vi "写入消息.vi"(8 "error in (no error)":errorcluster caption="错误输入（无错误）", 10 "操作者框架:消息待入队列":refnum<class "Message Enqueuer.lvclass">, 11 "用户操作输入":refnum<class "用户操作.lvclass">) -> (0 "error out":errorcluster caption="错误输出", 3 "用户操作输出":refnum<class "用户操作.lvclass">)   [LabVIEW 2020, in "用户操作.lvlib" / "用户操作.lvclass"]
uses:
  <vilib>/ActorFramework/Message Enqueuer/Message Enqueuer.lvclass
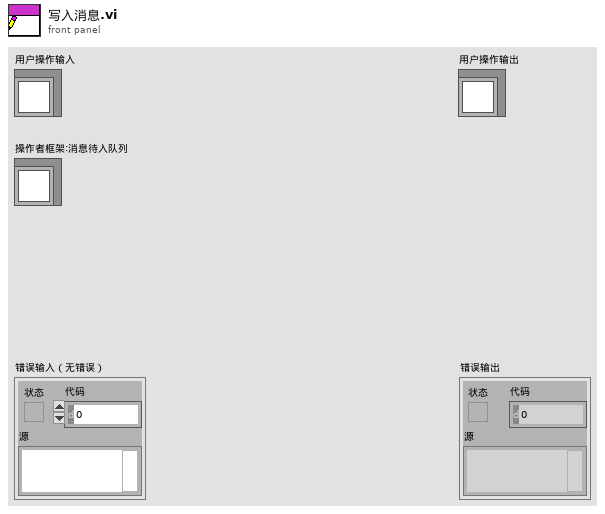
[diagram p1: front panel]
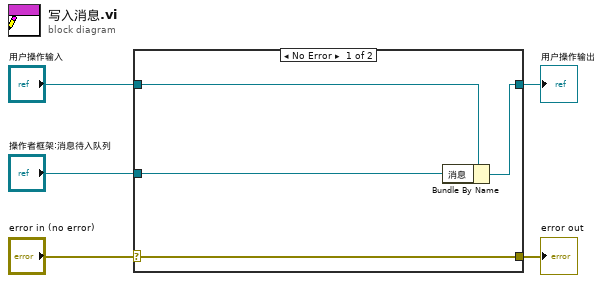
[diagram p0: block diagram]
diagram:
  n1 = case shown="No Error" "error in (no error)" {
    selector: "error in (no error)" -> [w9 w10]
    tunnel: [w9 w10] -> w4
    tunnel: [w7 w11] -> w2
    tunnel: "用户操作输入" -> [w8 w11]
    tunnel: "操作者框架:消息待入队列" -> [w6 _]
    frame No Error {
      n2 = Bundle By Name(cluster=w8, "消息"=w6) -> (w7:refnum<class "用户操作.lvclass">)
    }
    frame Error {
    }
  }
  "error out" <- w4
  "用户操作输出" <- w2
